vi "Lead Durability v2.vi"() -> ()   [LabVIEW 2013]
uses:
  <vilib>/Instr/_visa.llb/VISA Configure Serial Port (Serial Instr).vi
  <vilib>/Utility/file.llb/Write To Spreadsheet File (I64).vi
  <vilib>/express/express shared/transition.llb/Dynamic To Waveform Array.vi
  <vilib>/express/express signal manip/GetorSetDDTAttributes/Set DDT Attributes/SetT0.vi
  <vilib>/express/express shared/transition.llb/Waveform Array To Dynamic.vi
  <vilib>/express/express signal manip/GetorSetDDTAttributes/Set DDT Attributes/Set DDT Properties.xnode
panel:
  in  "initial reps":i32[](array[numeric])
  in  "Filename Suffix":string="test"
  in  "Stop if fail":bool
  in  "channel names":string[](array[string])
  in  "Reset 11":bool
  in  "Reset 10":bool
  in  "Reset 9":bool
  in  "Reset 8":bool
  in  "Reset 7":bool
  in  "Reset 6":bool
  in  "Reset 5":bool
  in  "Reset 4":bool
  in  "Reset 3":bool
  in  "Reset 2":bool
  in  "Reset 1":bool
  in  "Reset 0":bool
  out "green":i32[](array[numeric])
  out "Waveform Graph":i32[][](graph)
  in  "Play Button":bool
  out "Lead Contact":bool[](array[boolean])
  out "error out":errorcluster
  out "accel":string
  in  "Angle":dbl=180.0 min=0.0 max=350.0 step=5.0
  out "concatenated string 2":string
  out "concatenated string":string
  in  "Hz":dbl=2.0 min=0.25 max=2.5 step=0.25
  in  "stop":bool
  # "Initial Reps"
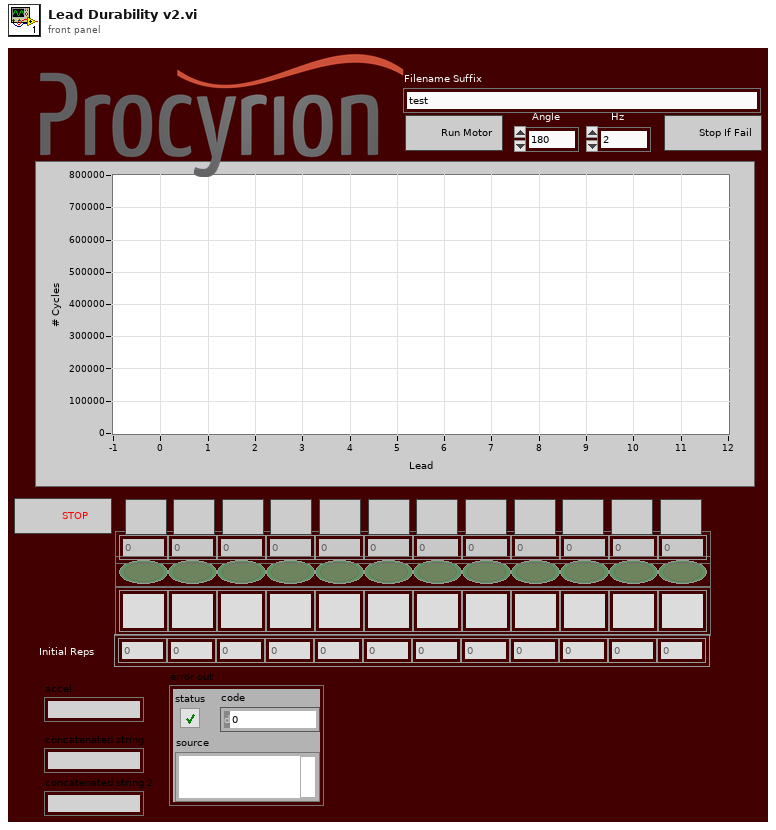
[diagram p1: front panel]
types:
  T1 = enum8{"Enabled", "Disabled", "Disabled and Grayed Out"}
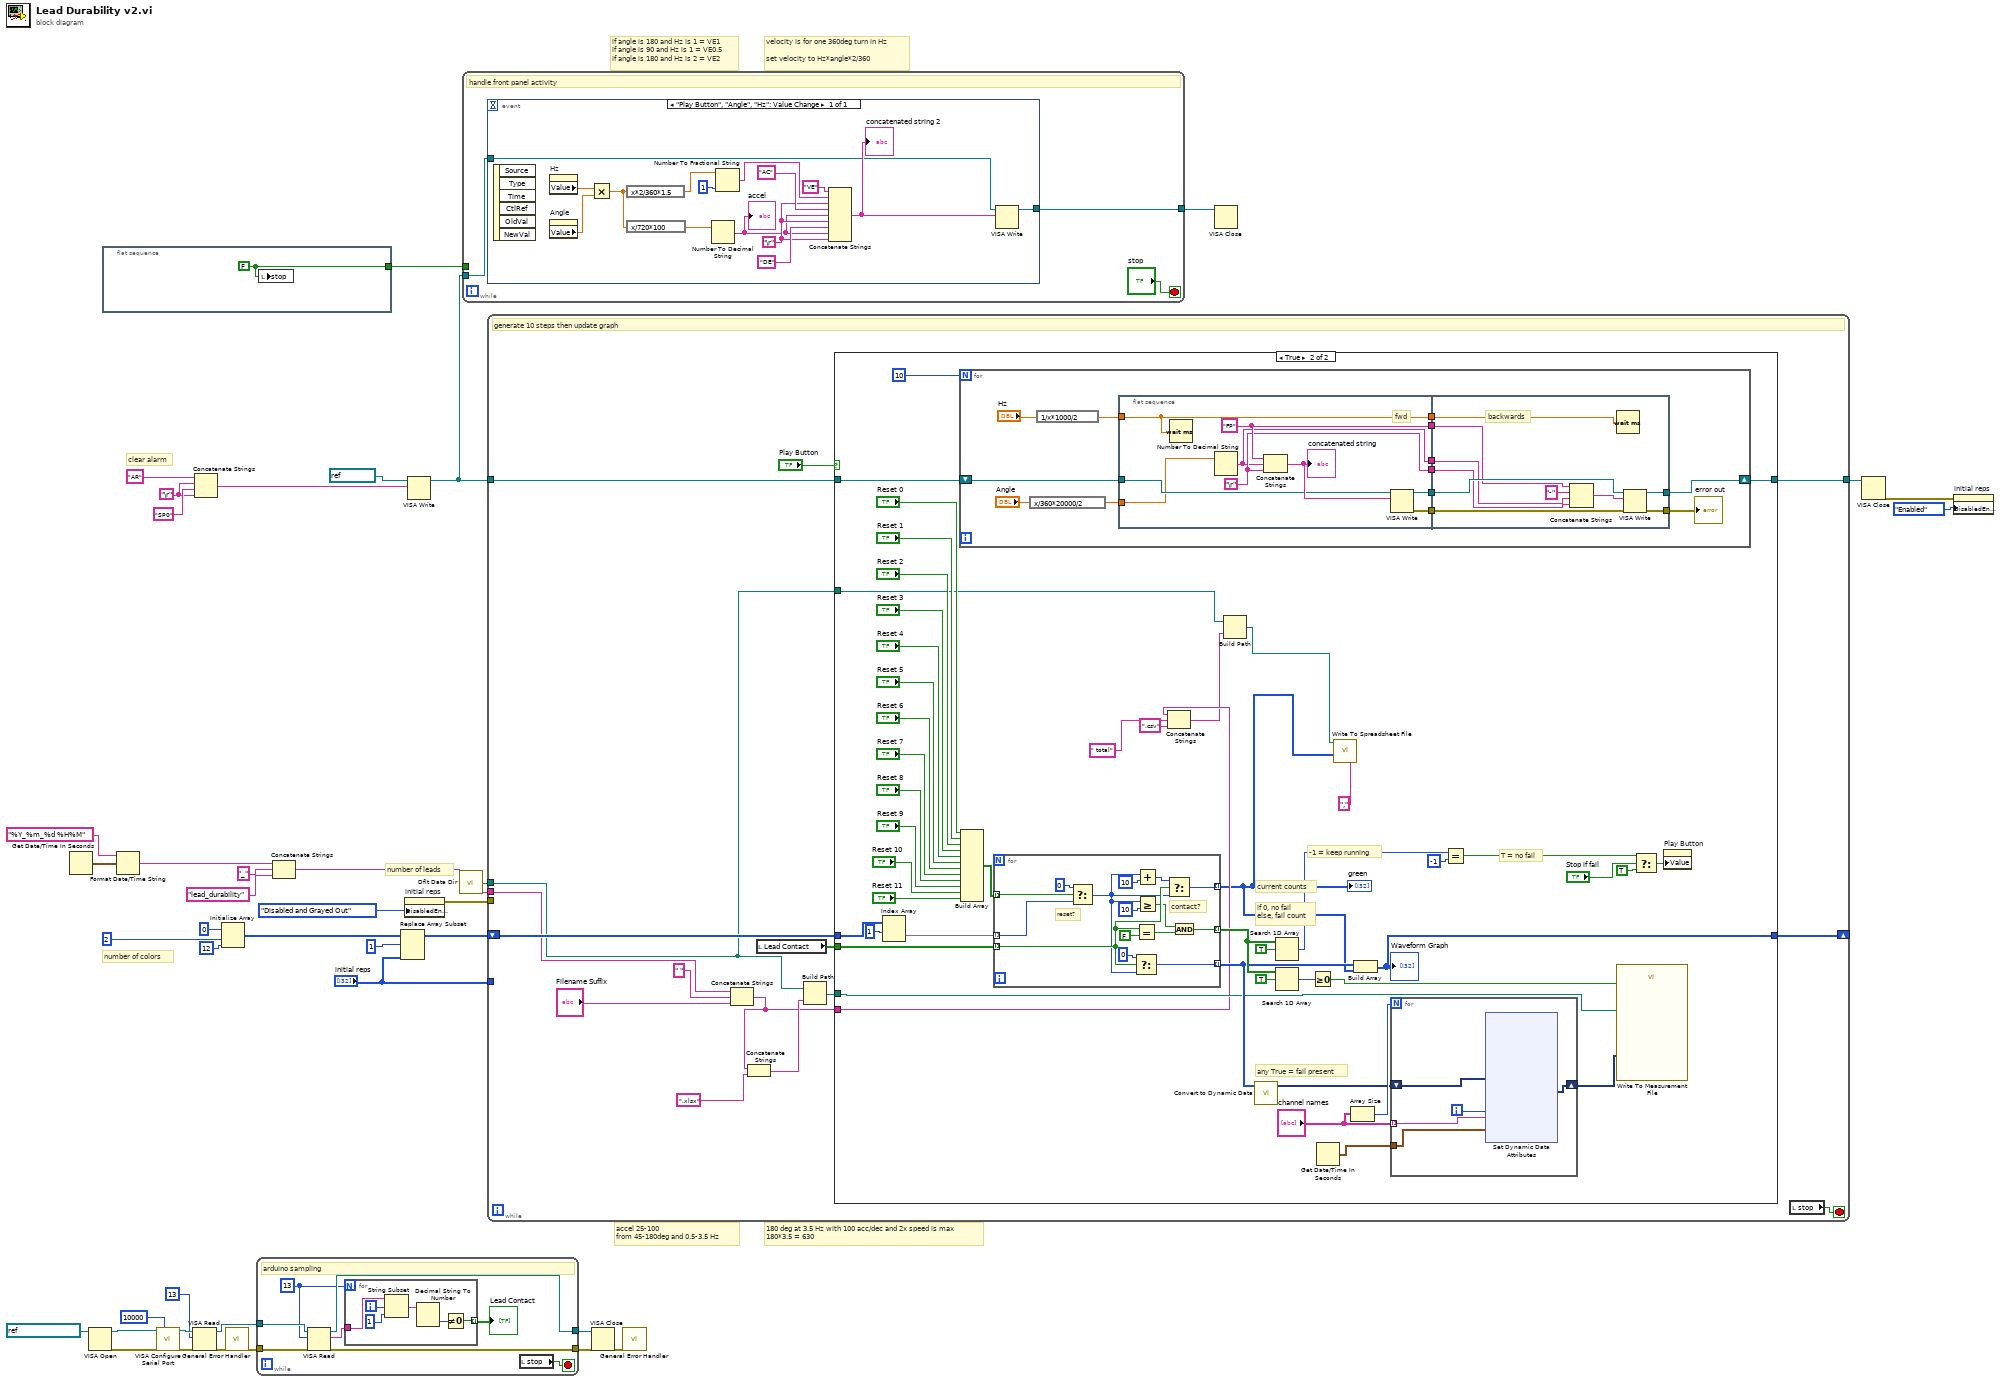
[diagram p0: block diagram]
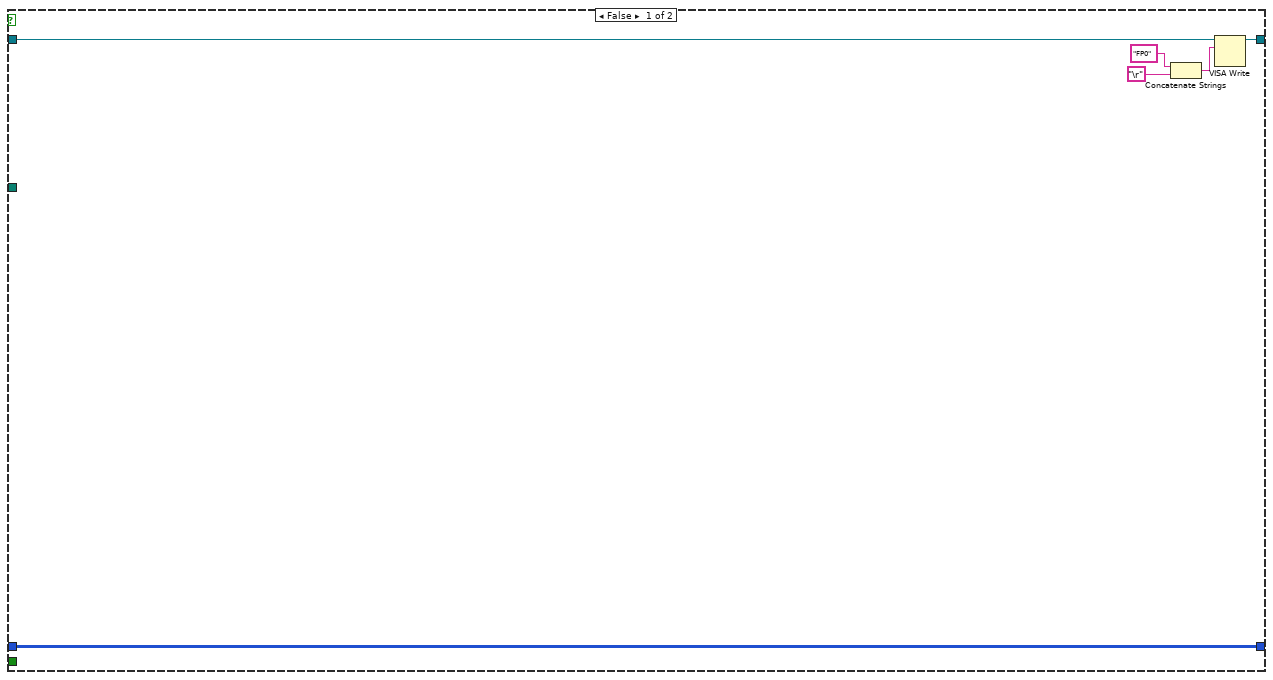
[diagram p2: hidden frame]
diagram:
  w36 = "\r"
  # "number of colors"
  # "number of leads"
  # "180 deg at 3.5 Hz with 100 acc/dec and 2x speed is max\n180*3.5 = 630"
  # "accel 25-100\nfrom 45-180deg and 0.5-3.5 Hz"
  # "if angle is 180 and Hz is 1 = VE1\nif angle is 90 and Hz is 1 = VE0.5\nif angle is 180 and Hz is 2 = VE2"
  # "velocity is for one 360deg turn in Hz\n\nset velocity to Hz*angle*2/360"
  # "clear alarm"
  n1 = Get Date/Time In Seconds() -> (seconds since 1Jan1904=w18:timestamp)
  n2 = VISA Open(VISA resource name=refnum<visa-resource-name> "ASRL8::INSTR" ("VISA resource")) -> (VISA resource name=w12:refnum<visa-resource-name>, error out=w11:errorcluster)  [unwired: 4 in]
  n3 = flat-sequence {
    tunnel: [w41] -> w32
    frame #0 {
      w41 = FALSE ("stop")
      n4 = local write "stop"(w41) -> ()
    }
  }
  n5 = Format Date/Time String(time format string (%c)="%Y_%m_%d %H%M", seconds (now)=w18) -> (date/time string=w15:string)  [unwired: 1 in]
  n6 = call-poly "VISA Configure Serial Port"("VISA resource name"=w12, "timeout (10sec)"=u32 10000, "error in (no error)"=w11) -> ("VISA resource name out"=w24:refnum<visa-resource-name>, "error out"=w23:errorcluster)  [unwired: 11 in]
  n7 = VISA Read(VISA resource name=w24, byte count=u32 13, error in (no error)=w23) -> (VISA resource name out=w22:refnum<visa-resource-name>, error out=w21:errorcluster)  [unwired: 2 out]
  n8 = Concatenate Strings("AR" ("write buffer"), w36, "SP0" ("write buffer"), w36) -> (w39:string)
  n9 = Initialize Array(0, 2 ("dimension size"), 12 ("dimension size")) -> (w7:i32[][])
  n10 = call <vilib>:"General Error Handler.vi"("error in (no error)"=w21) -> ("error out"=w14:errorcluster)  [unwired: 10 in, 4 out]
  n11 = while {
    tunnel: w22 -> [w47]
    tunnel: [w46] -> w28
    tunnel: w14 -> [w45]
    tunnel: [w42] -> w27
    stop <- w49 stop-if-true
    w43 = u32 13 ("byte count")
    # "arduino sampling"
    n12 = VISA Read(VISA resource name=w47, byte count=w43, error in (no error)=w45) -> (VISA resource name out=w46:refnum<visa-resource-name>, read buffer=w44:string, error out=w42:errorcluster)  [unwired: 1 out]
    n13 = for {
      N: w43 -> [_]
      tunnel: [w50] -> w48 mode=indexing
      tunnel: w44 -> [w55]
      i -> [w54]
      n14 = String Subset(string=w55, offset (0)=w54, length (rest)=1 ("length (rest)")) -> (substring=w52:string)
      n15 = Decimal String To Number(string=w52) -> (number=w51:i32)  [unwired: 2 in, 1 out]
      n16 = Not Equal To 0?(x=w51) -> (x != 0?=w50:bool)
    }
    "Lead Contact" <- w48
    n17 = local read "stop"() -> (w49:bool)
  }
  n18 = Concatenate Strings(w15, "_", "lead_durability" ("string")) -> (w10:string)
  n19 = Replace Array Subset(array=w7, new element="initial reps", index (row)=1) -> (w4:i32[][])  [unwired: 1 in]
  n20 = property on="initial reps" class="Arr (strict)"("DisabledEnum"=T1."Disabled and Grayed Out" ("Disabled")) -> (error out=w8:errorcluster)  [unwired: 2 in, 1 out]
  n21 = VISA Write(VISA resource name=refnum<visa-resource-name> "COM4", write buffer=w39) -> (VISA resource name out=w35:refnum<visa-resource-name>)  [unwired: 1 in, 2 out]
  n22 = call <vilib>:"Dflt Data Dir.vi"() -> ("App:Default Data Directory"=w1:path)
  n23 = while {
    tunnel: w35 -> [w57]
    tunnel: [w56] -> w33
    tunnel: w32 -> [_]
    stop <- "stop" stop-if-true
    # "handle front panel activity"
    n24 = event shown="[0] \"Play Button\", \"Angle\", \"Hz\": Value Change" {
      selector: _ -> [_]
      dyn-events: _ -> [_]
      timeout: _ -> [_]
      tunnel: w57 -> [w68]
      tunnel: [w59] -> w56
      event "Play Button", "Angle", "Hz": Value Change {
        w63 = "\r"
        n25 = event-data() -> ()  [unwired: 1 in, 6 out]
        n26 = property on="Hz" class="DigNum (strict)"() -> ("Value"=w61:dbl)  [unwired: 2 in, 2 out]
        n27 = property on="Angle" class="DigNum (strict)"() -> ("Value"=w60:dbl)  [unwired: 2 in, 2 out]
        n28 = Multiply(x=w61, y=w60) -> (x*y=w66:dbl)
        n29 = expression code="x*2/360*1.5"(w66) -> (w73:dbl)
        n30 = expression code="x/720*100"(w66) -> (w65:dbl)
        n31 = Number To Decimal String(number=w65) -> (decimal integer string=w62:string)  [unwired: 1 in]
        "accel" <- w62
        n32 = Number To Fractional String(number=w73, precision (6)=i16 1) -> (F-format string=w72:string)  [unwired: 2 in]
        n33 = Concatenate Strings("VE" ("write buffer"), w72, w63, "AC" ("write buffer"), w62, w63, "DE" ("write buffer"), w62, w63) -> (w69:string)
        "concatenated string 2" <- w69
        n34 = VISA Write(VISA resource name=w68, write buffer=w69) -> (VISA resource name out=w59:refnum<visa-resource-name>)  [unwired: 1 in, 2 out]
      }
    }
  }
  n35 = while {
    tunnel: w35 -> [w87]
    tunnel: [w88] -> w34
    shift-right: [w85] -> _
    shift-left: w4 -> [w83]
    tunnel: w10 -> [w81]
    tunnel: w8 -> [_]
    tunnel: "initial reps" -> [_]
    tunnel: w1 -> [w74]
    stop <- w86 stop-if-true
    # "generate 10 steps then update graph"
    n36 = Concatenate Strings(w81, " " ("string"), "Filename Suffix") -> (w75:string)
    n37 = Concatenate Strings(w75, ".xlsx" ("string")) -> (w77:string)
    n38 = local read "Lead Contact"() -> (w84:bool[])
    n39 = Build Path(base path=w74, name or relative path=w77) -> (appended path=w78:path)
    n40 = case shown="True" "Play Button" {
      tunnel: [w92 w141] -> w88
      tunnel: w87 -> [w93 w140]
      tunnel: w84 -> [_ w138]
      tunnel: [w94 w121] -> w85
      tunnel: w83 -> [w94 w136]
      tunnel: w78 -> [_ w104]
      tunnel: w75 -> [_ w102]
      tunnel: w74 -> [_ w98]
      frame False {
        n41 = Concatenate Strings("FP0" ("write buffer"), "\r") -> (w89:string)
        n42 = VISA Write(VISA resource name=w93, write buffer=w89) -> (VISA resource name out=w92:refnum<visa-resource-name>)  [unwired: 1 in, 2 out]
      }
      frame True {
        # "if 0, no fail\nelse, fail count"
        # "current counts"
        # "-1 = keep running"
        # "any True = fail present"
        # "T = no fail"
        n43 = Index Array(array=w136, index (row)=1) -> (element=w135:i32[])  [unwired: 1 in]
        n44 = for {
          N: 10 -> [_]
          shift-right: [w187] -> w141
          shift-left: w140 -> [w184]
          n45 = expression code="x/360*20000/2"("Angle") -> (w179:dbl)
          n46 = expression code="1/x*1000/2"("Hz") -> (w190:dbl)
          n47 = flat-sequence {
            tunnel: w190 -> [w200]
            tunnel: [w200] -> w189
            tunnel: w179 -> [w197]
            tunnel: w184 -> [w198]
            tunnel: [w196] -> w188
            tunnel: [w195] -> w185
            tunnel: [w194] -> w183
            tunnel: [w193] -> w182
            tunnel: [w192] -> w181
            tunnel: w189 -> [w210]
            tunnel: w188 -> [w209]
            tunnel: [w208] -> w187
            tunnel: [w207] -> w186
            tunnel: w185 -> [w206]
            tunnel: w183 -> [w205]
            tunnel: w182 -> [w204]
            tunnel: w181 -> [w203]
            frame #0 {
              w193 = "\r"
              w194 = "FP" ("write buffer")
              # "fwd"
              n48 = Wait (ms)(milliseconds to wait=w200) -> ()  [unwired: 1 out]
              n49 = Number To Decimal String(number=w197) -> (decimal integer string=w192:string)  [unwired: 1 in]
              n50 = Concatenate Strings(w194, w192, w193) -> (w199:string)
              "concatenated string" <- w199
              n51 = VISA Write(VISA resource name=w198, write buffer=w199) -> (VISA resource name out=w196:refnum<visa-resource-name>, error out=w195:errorcluster)  [unwired: 1 in, 1 out]
            }
            frame #1 {
              # "backwards"
              n52 = Concatenate Strings(w205, "-" ("string"), w203, w204) -> (w201:string)
              n53 = Wait (ms)(milliseconds to wait=w210) -> ()  [unwired: 1 out]
              n54 = VISA Write(VISA resource name=w209, write buffer=w201, error in (no error)=w206) -> (VISA resource name out=w208:refnum<visa-resource-name>, error out=w207:errorcluster)  [unwired: 1 out]
            }
          }
          "error out" <- w186
        }
        n55 = Build Array("Reset 0", "Reset 1", "Reset 2", "Reset 3", "Reset 4", "Reset 5", "Reset 6", "Reset 7", "Reset 8", "Reset 9", "Reset 10", "Reset 11") -> (w122:bool[])
        n56 = for {
          tunnel: w138 -> [w171] mode=indexing
          tunnel: w135 -> [w173] mode=indexing
          tunnel: [w177] -> w99 mode=indexing
          tunnel: [w164] -> w108 mode=indexing
          tunnel: w122 -> [w174] mode=indexing
          tunnel: [w165] -> w112 mode=indexing
          # "contact?"
          # "reset?"
          n57 = Select(t=0, s=w174, f=w173) -> (s? t:f=w169:i32)
          n58 = Equal?(x=w171, y=FALSE) -> (x = y?=w166:bool)
          n59 = Select(t=0, s=w171, f=w169) -> (s? t:f=w164:i32)
          n60 = Add(x=w169, y=10) -> (x+y=w178:i32)
          n61 = Greater Or Equal?(x=w169, y=10) -> (x >= y?=w167:bool)
          n62 = Select(t=w178, s=w171, f=w169) -> (s? t:f=w177:i32)
          n63 = And(x=w167, y=w166) -> (x .and. y?=w165:bool)
        }
        "green" <- w99
        n64 = Concatenate Strings(w102, " total" ("name or relative path"), ".csv" ("string")) -> (w101:string)
        n65 = Build Path(base path=w98, name or relative path=w101) -> (appended path=w100:path)
        n66 = call "Convert to Dynamic Data"("Array"=w108) -> ("Dynamic Data Type"=w107:dynamicdata)  [unwired: 3 in]
        n67 = Search 1D Array(1D array=w112, element=TRUE) -> (index of element=w118:i32)  [unwired: 1 in]
        n68 = Search 1D Array(1D array=w112, element=TRUE) -> (index of element=w110:i32)  [unwired: 1 in]
        n69 = Greater Or Equal To 0?(x=w110) -> (x >= 0?=w109:bool)
        n70 = Get Date/Time In Seconds() -> (seconds since 1Jan1904=w95:timestamp)
        n71 = call-poly <vilib>:"Write To Spreadsheet File.vi"("delimiter (\\t)"="," ("delimiter (\\t)"), "1D data"=w99, "file path (dialog if empty)"=w100) -> ()  [unwired: 5 in, 1 out]
        n72 = Array Size(array="channel names") -> (size(s)=w113:i32)
        n73 = Build Array(w108, w99) -> (w121:i32[][])
        "Waveform Graph" <- w121
        n74 = for {
          N: w113 -> [_]
          tunnel: "channel names" -> [w146] mode=indexing
          shift-right: [w143] -> w106
          shift-left: w107 -> [w145]
          tunnel: w95 -> [w142]
          i -> [w144]
          n75 = xnode "Set Dynamic Data Attributes"("Signals In"=w145, "Signal Index"=w144, "Signal Name"=w146, "Timestamp"=w142) -> ("Signals Out"=w143:dynamicdata)  [unwired: 1 in, 1 out]
        }
        n76 = Equal?(x=w118, y=-1) -> (x = y?=w116:bool)
        n77 = call "Write To Measurement File"("Signals"=w106, "Enable"=w109, "Filename"=w104) -> ()  [unwired: 14 in, 3 out]
        n78 = Select(t=w116, s="Stop if fail", f=TRUE) -> (s? t:f=w114:bool)
        n79 = property on="Play Button" class="Bool (strict)"("Value"=w114) -> ()  [unwired: 2 in, 2 out]
      }
    }
    n80 = local read "stop"() -> (w86:bool)
  }
  n81 = VISA Close(VISA resource name=w28, error in (no error)=w27) -> (error out=w26:errorcluster)
  n82 = call <vilib>:"General Error Handler.vi"("error in (no error)"=w26) -> ()  [unwired: 10 in, 5 out]
  n83 = VISA Close(VISA resource name=w33) -> ()  [unwired: 1 in, 1 out]
  n84 = VISA Close(VISA resource name=w34) -> (error out=w2:errorcluster)  [unwired: 1 in]
  n85 = property on="initial reps" class="Arr (strict)"(error in=w2, "DisabledEnum"=T1."Enabled" ("Disabled")) -> ()  [unwired: 1 in, 2 out]
